vi "Write Timeout Delivery Notifier.vi"(8 "error in (no error)":errorcluster, 10 "Timeout Delivery Notifier":refnum<notifier>, 11 "_State Machine Actor in":refnum<class "_State Machine Actor.lvclass">) -> (0 "error out":errorcluster, 3 "_State Machine Actor out":refnum<class "_State Machine Actor.lvclass">)   [LabVIEW 2024]
uses:
  _State Machine Actor.lvclass/_State Machine Actor.ctl
  _State Machine Actor.lvclass
  C:/Program Files (x86)/National Instruments/LabVIEW 2024/vi.lib/ActorFramework/Actor/Actor.lvclass
  C:/Users/uspoaotto/OneDrive - Oregon Tool/Desktop/working copies/stateMachineActor/src/_State Machine Actor/_State Machine Actor/_State Machine Actor.lvclass
  <vilib>/ActorFramework/Time-Delayed Send Message/Time-Delay Override Options.ctl
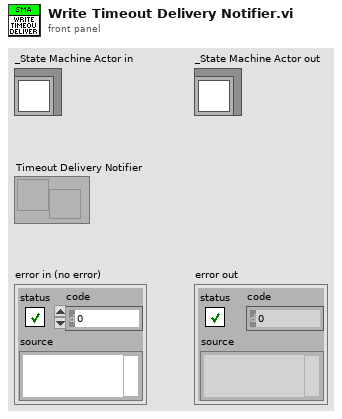
[diagram p1: front panel]
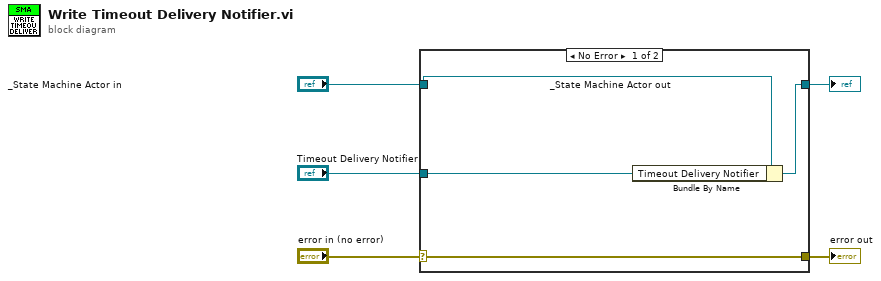
[diagram p0: block diagram]
diagram:
  n1 = case shown="No Error" "error in (no error)" {
    selector: "error in (no error)" -> [w9 w10]
    tunnel: [w9 w10] -> w4
    tunnel: [w7 w11] -> w2
    tunnel: "_State Machine Actor in" -> [w8 w11]
    tunnel: "Timeout Delivery Notifier" -> [w6 _]
    frame No Error {
      n2 = Bundle By Name(cluster=w8, "Timeout Delivery Notifier"=w6) -> (w7:refnum<class "_State Machine Actor.lvclass">)
    }
    frame Error {
    }
  }
  "error out" <- w4
  "_State Machine Actor out" <- w2
